vi "互相关分析.vi"() -> ()   [LabVIEW 2019]
uses:
  <vilib>/Analysis/2dsp.llb/1D Cross Correlation (DBL).vi
  <vilib>/Analysis/NI_AALBase.lvlib
  <vilib>/Analysis/NI_AALPro.lvlib
panel:
  out "相关后波形":cluster{i32, dbl, "Rxy":dbl[]}(graph)
  out "信号波形":cluster{i32, dbl, dbl[][]}(graph)
  in  "采样频率":dbl format="%#_13g"
  in  "初始相位2":dbl format="%#_13g"
  in  "频率2":dbl format="%#_13g"
  in  "初始相位1":dbl format="%#_13g"
  in  "频率1":dbl format="%#_13g"
  in  "采样点数":dbl format="%#_13g"
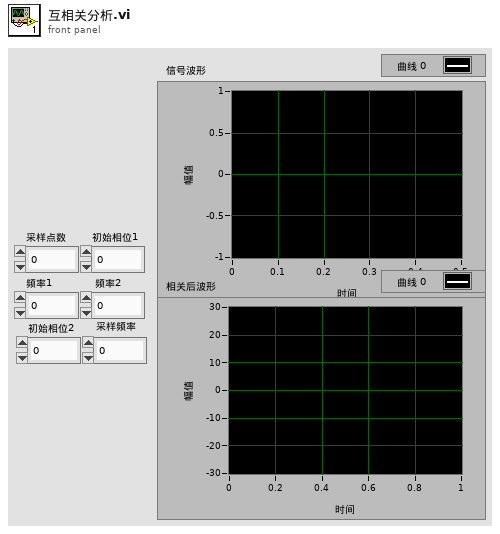
[diagram p1: front panel]
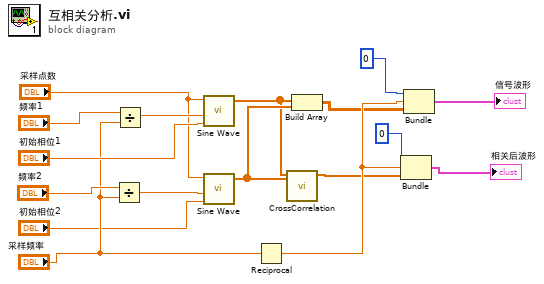
[diagram p0: block diagram]
diagram:
  n1 = Divide(x="频率2", y="采样频率") -> (x/y=w8:dbl)
  n2 = Divide(x="频率1", y="采样频率") -> (x/y=w12:dbl)
  n3 = call <vilib>:"Sine Wave.vi"("samples"="采样点数", "frequency"=w12, "phase in"="初始相位1") -> ("sine wave"=w5:dbl[])  [unwired: 2 in, 2 out]
  n4 = call <vilib>:"Sine Wave.vi"("samples"="采样点数", "frequency"=w8, "phase in"="初始相位2") -> ("sine wave"=w6:dbl[])  [unwired: 2 in, 2 out]
  n5 = Reciprocal(x="采样频率") -> (1/x=w17:dbl)
  n6 = call-poly <vilib>:"CrossCorrelation.vi"("Y"=w6, "X"=w5) -> ("Rxy"=w3:dbl[])  [unwired: 8 in, 1 out]
  n7 = Build Array(w5, w6) -> (w4:dbl[][])
  n8 = Bundle(0, w17, "Rxy"=w3) -> (→"相关后波形":cluster{i32, dbl, "Rxy":dbl[]})  [unwired: 1 in]
  n9 = Bundle(0, w17, w4) -> (→"信号波形":cluster{i32, dbl, dbl[][]})  [unwired: 1 in]
